vi "ecu_fgv.vi"(7 "mode":enum16{"read", "write"}(ring), 8 "error in (no error)":errorcluster, 11 "data in":T1) -> (0 "error out":errorcluster, 3 "data out":T1)   [LabVIEW 2019]
uses:
  gui/ecu_dataCluster.ctl
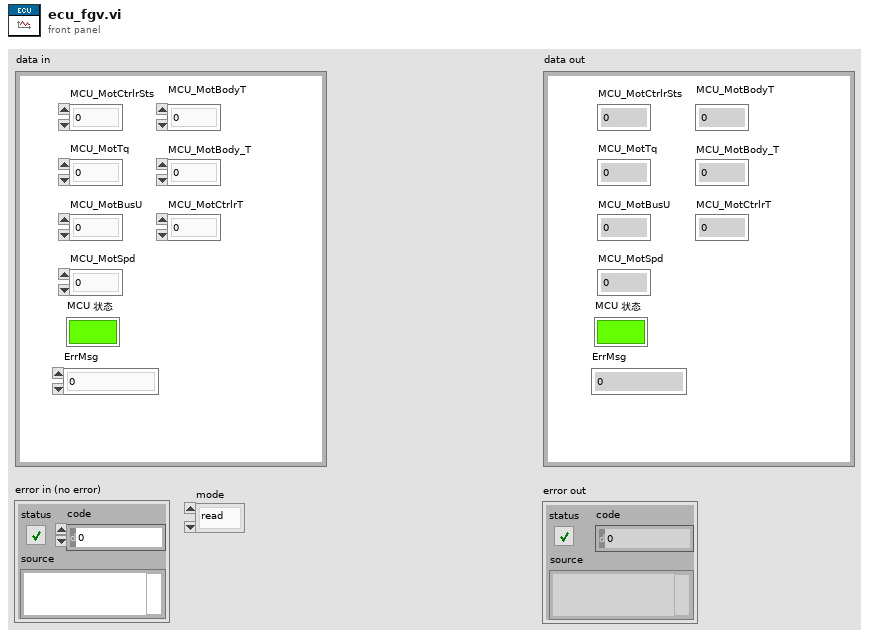
[diagram p1: front panel]
types:
  T1 = typedef "ecu_dataCluster.ctl" = cluster{"MCU_MotCtrlrSts":dbl, "MCU_MotTq":dbl, "MCU_MotBusU":dbl, "MCU_MotSpd":dbl, "MCU_MotBodyT":dbl, "MCU_MotBody_T":dbl, "MCU_MotCtrlrT":dbl, "MCU 状态":bool, "ErrMsg":i64}
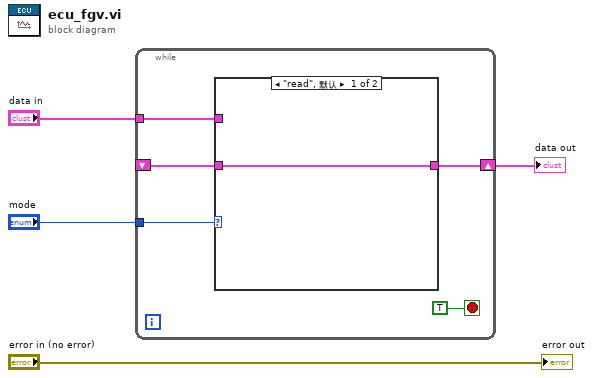
[diagram p0: block diagram]
diagram:
  n1 = while {
    tunnel: "mode" -> [w9]
    tunnel: "data in" -> [w8]
    shift-right: [w7] -> w2
    shift-left: _ -> [w6]
    stop <- TRUE stop-if-true
    n2 = case shown="\"read\", 默认" w9 {
      tunnel: [w10 w11] -> w7
      tunnel: w8 -> [_ w11]
      tunnel: w6 -> [w10 _]
      frame "read", Default {
      }
      frame "write" {
      }
    }
  }
  "data out" <- w2
  "error out" <- "error in (no error)"
